vi "Get Timeout Property Name.vi"() -> ()   [LabVIEW 2017]
panel:
  out "Property Name":string="Async Init Timeout"
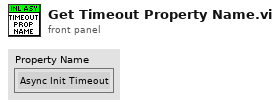
[diagram p1: front panel]
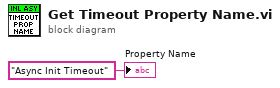
[diagram p0: block diagram]
diagram:
  "Property Name" <- "Async Init Timeout"
